vi "Scope_Cap_meas.vi"(0 "VISA resource name":refnum<visa-resource-name>="USB0::0x0699::0x0522::C019376::INSTR", 1 "file path (dialog if empty)":path=path "D:/Projects/C2000/Grande/Data/System/Cap/New", 5 "string":string="B11_ALT", 7 "Frequency/Sample Rate/Bandwidth (Hz or Sa/s)":dbl, 11 "error in (no error)":errorcluster, 13 "Resistance":dbl=1004.1 format="%#_13g", 14 "Condition":string="NO_device") -> (3 "Path_out":path=path "D:/Projects/C2000/Grande/Data/System/Cap/Waveform/B11_ALT_NO_device_CH1.txt", 8 "Cap":dbl=2.575167290815062e-11 format="%#_6p", 15 "error out":errorcluster)   [LabVIEW 2019]
uses:
  <userlib>/_TI-LA/Instr Drivers/Signal Generator/3352x/Driver/EasyIO/Typedef/Channel.ctl
  <userlib>/_TI-LA/Instr Drivers/Signal Generator/3352x/Driver/EasyIO/Typedef/Standard Waveform Settings.ctl
  <userlib>/_TI-LA/Instr Drivers/Signal Generator/3352x/Driver/EasyIO/Typedef/Waveform Function.ctl
  <userlib>/_TI-LA/Instr Drivers/Signal Generator/3352x/Driver/EasyIO/Typedef/Amplitude Settings.ctl
  <userlib>/_TI-LA/Instr Drivers/Signal Generator/3352x/Driver/EasyIO/Typedef/Amplitude Unit.ctl
  <userlib>/_TI-LA/Instr Drivers/Signal Generator/3352x/Driver/EasyIO/Typedef/Phase Configuration.ctl
  <userlib>/_TI-LA/Instr Drivers/Signal Generator/3352x/Driver/EasyIO/Typedef/Angle Unit.ctl
  <userlib>/_TI-LA/Instr Drivers/Oscilloscope/MSO5X/Driver/Base/Public/Data/Low Level/Fetch (Waveform).vi
  <vilib>/Waveform/WDTFileIO.llb/Export Waveform To Spreadsheet File.vi
  <userlib>/_TI-LA/Instr Drivers/Oscilloscope/MSO5X/Driver/Base/Tektronix MSO5X Series.lvlib
  <userlib>/_TI-LA/Instr Drivers/Oscilloscope/MSO5X/Driver/MSO5X.lvlib
  <vilib>/ptbypt/NI_PtbyPt.lvlib
  <userlib>/_TI-LA/Instr Drivers/Signal Generator/3352x/Driver/Base/Agilent 3352X Series.lvlib
  <userlib>/_TI-LA/Instr Drivers/Signal Generator/3352x/Driver/3352x.lvlib
  common/Comman_nilesh/File_Write/Data_Logging.lvclass
panel:
  in  "SG":refnum<visa-resource-name>="USB0::0x0957::0x1607::MY50001293::INSTR"
  out "Waveform Graph":waveform(dbl)[](graph)=[{"t0"=timestamp(1.5999999995698275e-10 s since 1904-01-01), "dt"=1.6e-10, "Y"=array[7000 elements]}, {"t0"=timestamp(1.5999999995698275e-10 s since 1904-01-01), "dt"=1.6e-10, "Y"=array[7000 elements]}]
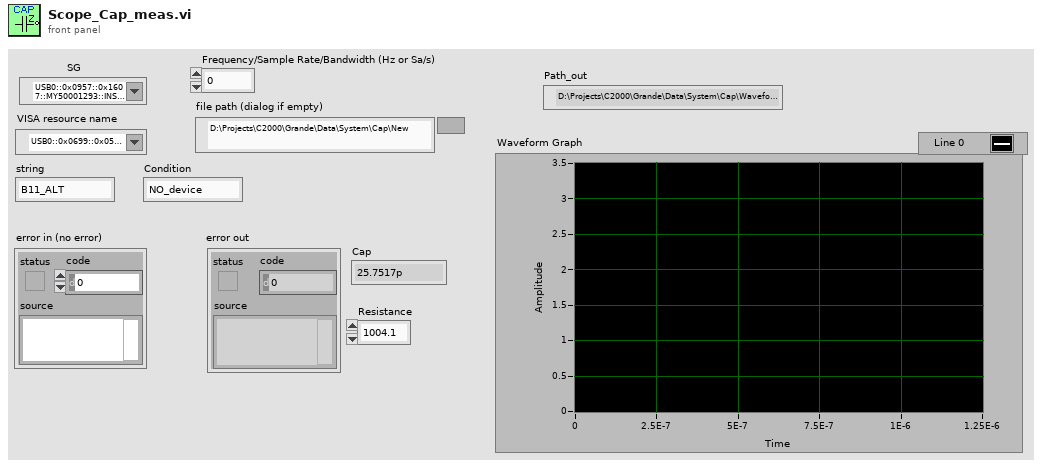
[diagram p1: front panel]
types:
  T1 = typedef "3352x.lvlib/Standard Waveform Settings.ctl" = cluster{"Waveform Function":T2, "Frequency/Sample Rate/Bandwidth (Hz or Sa/s)":dbl, "DC Offset (V)":dbl, "Amplitude Settings":T3, "Phase Settings":T5}
  T2 = typedef "3352x.lvlib/Waveform Function.ctl" = enum16{"Sine", "Square", "Ramp", "Noise", "DC", "Triangle", "Pulse", "Sinc", "D-Lorentz", "Gaussian", "Expo Fall", "Expo Rise", "Haversine"}
  T3 = typedef "3352x.lvlib/Amplitude Settings.ctl" = cluster{"Amplitude (100m)":dbl, "Amplitude Unit (VPP)":T4}
  T4 = typedef "3352x.lvlib/Amplitude Unit.ctl" = enum16{"VPP", "VRMS", "DBM"}
  T5 = typedef "3352x.lvlib/Phase Configuration.ctl" = cluster{"Phase Angle (Deg/Rad)":dbl, "Angle Unit":T6}
  T6 = typedef "3352x.lvlib/Angle Unit.ctl" = enum16{"Degree", "Radian", "Second"}
  T7 = typedef "3352x.lvlib/Channel.ctl" = enum16{"1", "2"}
  T8 = enum16{"Numeric", "High Z", "Minimum", "Maximum", "Default"}
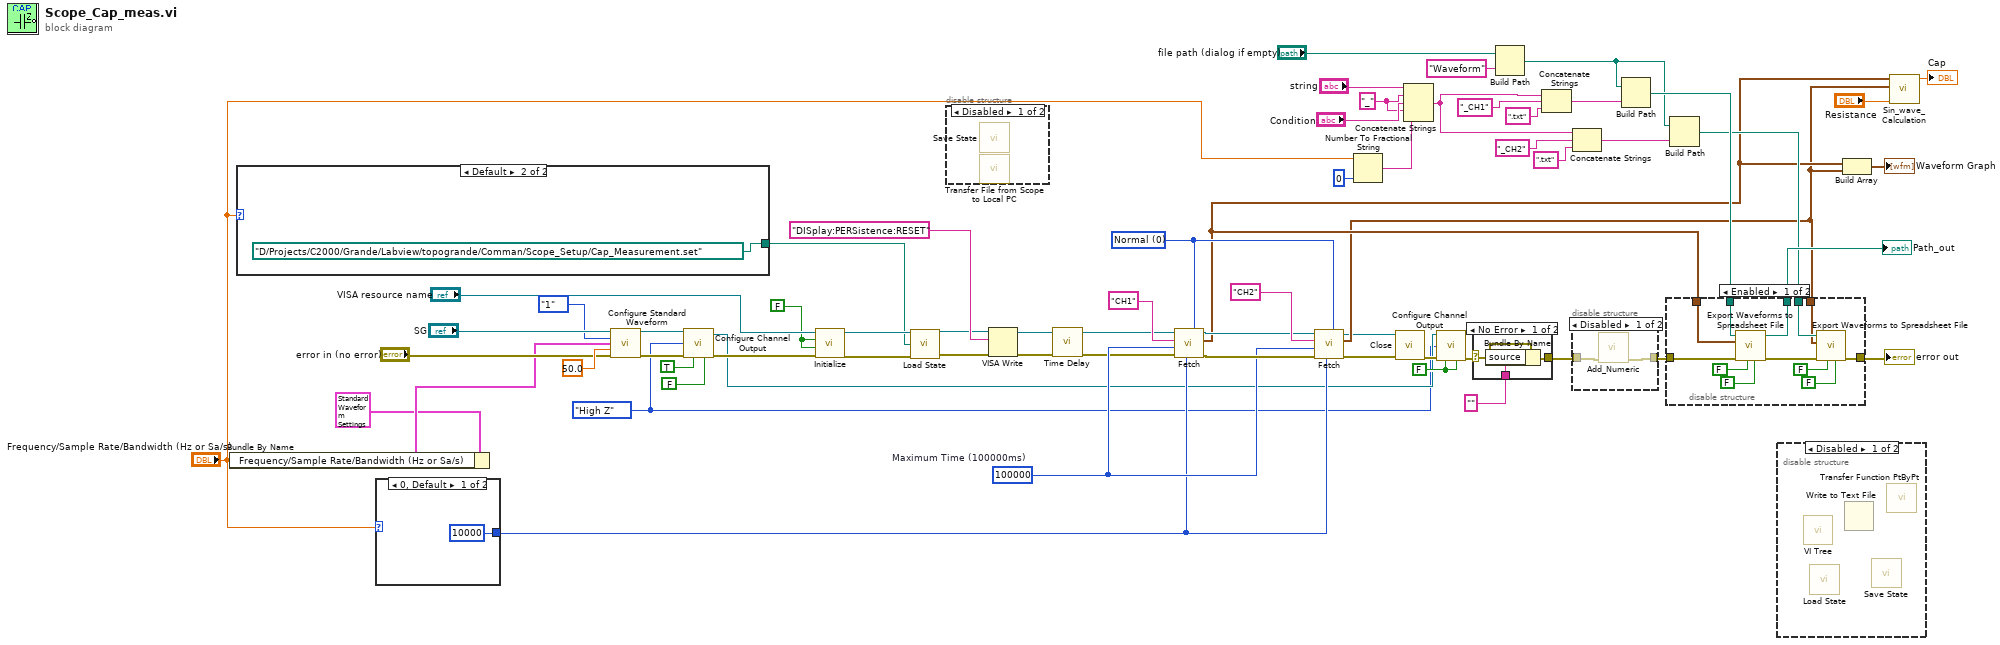
[diagram p0: block diagram]
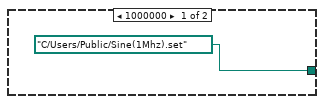
[diagram p3: hidden frame]
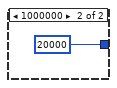
[diagram p4: hidden frame]
diagram:
  w3 = FALSE ("Enable Output (T: Enable)")
  w1 = T8."High Z" ("Output Impedence Mode (0: Numeric)")
  w11 = "_"
  w46 = u32 100000  # Maximum Time (100000ms)
  w36 = u16 0 items=["Normal", "Came from a MATH"] ("Ref Waveform Type")
  w62 = FALSE ("Reset (True)")
  n1 = Bundle By Name(cluster=T1 {"Waveform Function"=enum."Sine", "Frequency/Sample Rate/Bandwidth (Hz or Sa/s)"=5000000.0, "DC Offset (V)"=1.65, "Amplitude Settings"={"Amplitude (100m)"=3.3, "Amplitude Unit (VPP)"=enum."VPP"}, "Phase Settings"={"Phase Angle (Deg/Rad)"=0.0, "Angle Unit"=enum."Degree"}} ("Standard Waveform Settings"), "Frequency/Sample Rate/Bandwidth (Hz or Sa/s)"="Frequency/Sample Rate/Bandwidth (Hz or Sa/s)") -> (w15:T1)
  n2 = case shown="Default" "Frequency/Sample Rate/Bandwidth (Hz or Sa/s)" {
    tunnel: [path "C:/Users/Public/Sine(1Mhz).set" ("File Path in PC (“C:\\File.set”)") path "D:/Projects/C2000/Grande/Labview/topogrande/Comman/Scope_Setup/Cap_Measurement.set" ("File Path in PC (“C:\\File.set”)")] -> w12
    frame 1000000 {
    }
    frame Default {
    }
  }
  n3 = case shown="0, Default" "Frequency/Sample Rate/Bandwidth (Hz or Sa/s)" {
    tunnel: [10000 ("Ending Point (2500)") 20000 ("Ending Point (2500)")] -> w13
    frame 0, Default {
    }
    frame 1000000 {
    }
  }
  n4 = call <userlib>:"Configure Standard Waveform.vi"("VISA resource name"="SG", "Channel"=Channel."1", "Standard Waveform Settings"=w15, "Duty Cycle (%)"=50.0, "error in"="error in (no error)") -> ("Dup VISA resource name"=w23:refnum<visa-resource-name>, "error out"=w24:errorcluster)  [unwired: 9 in]
  n5 = call <userlib>:"Configure Channel Output.vi"("VISA resource name"=w23, "Output Impedence Mode (0: Numeric)"=w1, "error in (no error)"=w24, "Enable Output (T: Enable)"=TRUE, "Enable Voltage Limit (T: Enable)"=FALSE) -> ("VISA resource name out"=w2:refnum<visa-resource-name>, "error out"=w16:errorcluster)  [unwired: 9 in]
  n6 = call <userlib>:"Initialize.vi"("error in (no error)"=w16, "Reset (True)"=w62, "ID Query (True)"=w62, "VISA resource name"="VISA resource name") -> ("error out"=w44:errorcluster, "VISA resource name out"=w45:refnum<visa-resource-name>)  [unwired: 6 in]
  n7 = call <userlib>:"Load State.vi"("VISA resource name"=w45, "File Path in PC (“C:\\File.set”)"=w12, "error in"=w44) -> ("VISA resource name out"=w39:refnum<visa-resource-name>, "error out"=w38:errorcluster)  [unwired: 11 in]
  n8 = disable-structure shown="Disabled" {
    frame Disabled {
      n9 = call <userlib>:"Save State.vi"() -> ()  [unwired: 14 in, 2 out]
      n10 = call <userlib>:"Transfer File from Scope to Local PC.vi"() -> ()  [unwired: 14 in, 2 out]
    }
    frame Enabled {
    }
  }
  n11 = VISA Write(VISA resource name=w39, write buffer="DISplay:PERSistence:RESET", error in (no error)=w38) -> (VISA resource name out=w37:refnum<visa-resource-name>, error out=w29:errorcluster)  [unwired: 1 out]
  n12 = call "Time Delay"("error in (no error)"=w29) -> ("error out"=w28:errorcluster)  [unwired: 10 in]
  n13 = call-poly <userlib>:"Fetch.vi"("Ref Waveform Type"=w36, "Ending Point (2500)"=w13, "error in (no error)"=w28, "Maximum Time (100000ms)"=w46, "Channel (CH1)"="CH1", "VISA resource name"=w37) -> ("error out"=w56:errorcluster, "Waveform Graph"=w35:waveform(dbl), "VISA resource name out"=w57:refnum<visa-resource-name>)  [unwired: 3 in]
  n14 = call-poly <userlib>:"Fetch.vi"("Ref Waveform Type"=w36, "Ending Point (2500)"=w13, "error in (no error)"=w56, "Maximum Time (100000ms)"=w46, "Channel (CH1)"="CH2", "VISA resource name"=w57) -> ("error out"=w30:errorcluster, "Waveform Graph"=w34:waveform(dbl), "VISA resource name out"=w31:refnum<visa-resource-name>)  [unwired: 3 in]
  n15 = Number To Fractional String(number="Frequency/Sample Rate/Bandwidth (Hz or Sa/s)", precision (6)=i16 0) -> (F-format string=w10:string)  [unwired: 2 in]
  n16 = call <userlib>:"Close.vi"("error in (no error)"=w30, "VISA resource name"=w31) -> ("error out"=w5:errorcluster)  [unwired: 9 in]
  n17 = Concatenate Strings("string", w11, "Condition", w11, w10) -> (w27:string)
  n18 = call <userlib>:"Configure Channel Output.vi"("VISA resource name"=w2, "Output Impedence Mode (0: Numeric)"=w1, "error in (no error)"=w5, "Enable Output (T: Enable)"=w3, "Enable Voltage Limit (T: Enable)"=w3) -> ("error out"=w4:errorcluster)  [unwired: 9 in, 1 out]
  n19 = case shown="No Error" w4 {
    selector: w4 -> [w71 w72]
    tunnel: "" -> [w70 _]
    tunnel: [w69 w72] -> w7
    frame No Error {
      n20 = Bundle By Name(cluster=w71, "source"=w70) -> (w69:errorcluster)
    }
    frame Error {
    }
  }
  n21 = Build Path(base path="file path (dialog if empty)", name or relative path="Waveform") -> (appended path=w49:path)
  n22 = Concatenate Strings(w27, "_CH1" ("string"), ".txt" ("name or relative path")) -> (w51:string)
  n23 = Concatenate Strings(w27, "_CH2" ("string"), ".txt" ("name or relative path")) -> (w48:string)
  n24 = disable-structure shown="Disabled" {
    disable-tunnel: w7 -> [w74 w75]
    disable-tunnel: [w73 w75] -> w6
    frame Disabled {
      n25 = call "Add_Numeric.vi"("Error In"=w74) -> ("error out"=w73:errorcluster)  [unwired: 13 in, 1 out]
    }
    frame Enabled {
    }
  }
  n26 = Build Path(base path=w49, name or relative path=w51) -> (appended path=w50:path)
  n27 = Build Path(base path=w49, name or relative path=w48) -> (appended path=w42:path)
  n28 = disable-structure shown="Enabled" {
    disable-tunnel: w6 -> [w85 w88]
    disable-tunnel: w50 -> [w84 _]
    disable-tunnel: [w80 w88] -> w47
    disable-tunnel: [w79 _] -> w43
    disable-tunnel: w42 -> [w78 _]
    disable-tunnel: w35 -> [w77 _]
    disable-tunnel: w34 -> [w76 _]
    frame Enabled {
      n29 = call-poly <vilib>:"Export Waveforms to Spreadsheet File.vi"("header? (write header:T)"=FALSE, "append to file? (new file:F)"=FALSE, "error in (no error)"=w85, "waveform"=w77, "file path (dialog if empty)"=w84) -> ("error out"=w81:errorcluster, "new file path (Not A Path if cancelled)"=w79:path)  [unwired: 5 in]
      n30 = call-poly <vilib>:"Export Waveforms to Spreadsheet File.vi"("header? (write header:T)"=FALSE, "append to file? (new file:F)"=FALSE, "error in (no error)"=w81, "waveform"=w76, "file path (dialog if empty)"=w78) -> ("error out"=w80:errorcluster)  [unwired: 5 in, 1 out]
    }
    frame Disabled {
    }
  }
  "error out" <- w47
  "Path_out" <- w43
  n31 = disable-structure shown="Disabled" {
    frame Disabled {
      n32 = call <userlib>:"VI Tree.vi"() -> ()  [unwired: 12 in]
      n33 = call <userlib>:"Load State.vi"() -> ()  [unwired: 14 in, 2 out]
      n34 = Write to Text File() -> ()  [unwired: 4 in, 3 out]
      n35 = call <userlib>:"Save State.vi"() -> ()  [unwired: 14 in, 2 out]
      n36 = call <vilib>:"Transfer Function PtByPt.vi"() -> ()  [unwired: 5 in, 4 out]
    }
    frame Enabled {
    }
  }
  n37 = Build Array(w35, w34) -> (→"Waveform Graph":waveform(dbl)[])
  n38 = call "Sin_wave_Calculation.vi"("Resistance"="Resistance", "CH2"=w34, "CH1"=w35) -> ("Cap"=→"Cap":dbl)  [unwired: 8 in]
